vi "configureAcquisition.vi"(6 "imagePaths":path[](array[path]), 7 "saveImages?":bool, 8 "error in (no error)":errorcluster, 9 "number of Images":i32, 10 "CamaraSettings":refnum<class "CamaraSettings.lvclass">, 11 "NetworkWinX32 in":refnum<class "NetworkWinX32.lvclass">) -> (0 "error out":errorcluster, 3 "NetworkWinX32 out":refnum<class "NetworkWinX32.lvclass">)   [LabVIEW 2011, in "Hardware.lvlib" / "HWControllers.lvlib" / "NetworkWinX32.lvclass"]
uses:
  NetworkWinX32.lvclass
  Tools/CameraSettings/CamaraSettings.lvclass
  NetworkWinX32.lvclass/NetworkWinX32.ctl
  Channels/Camera/WinX32_SA/WinX32Camera.lvclass
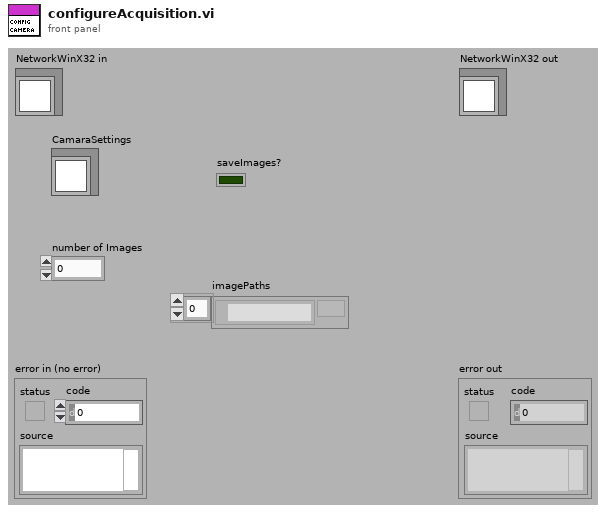
[diagram p1: front panel]
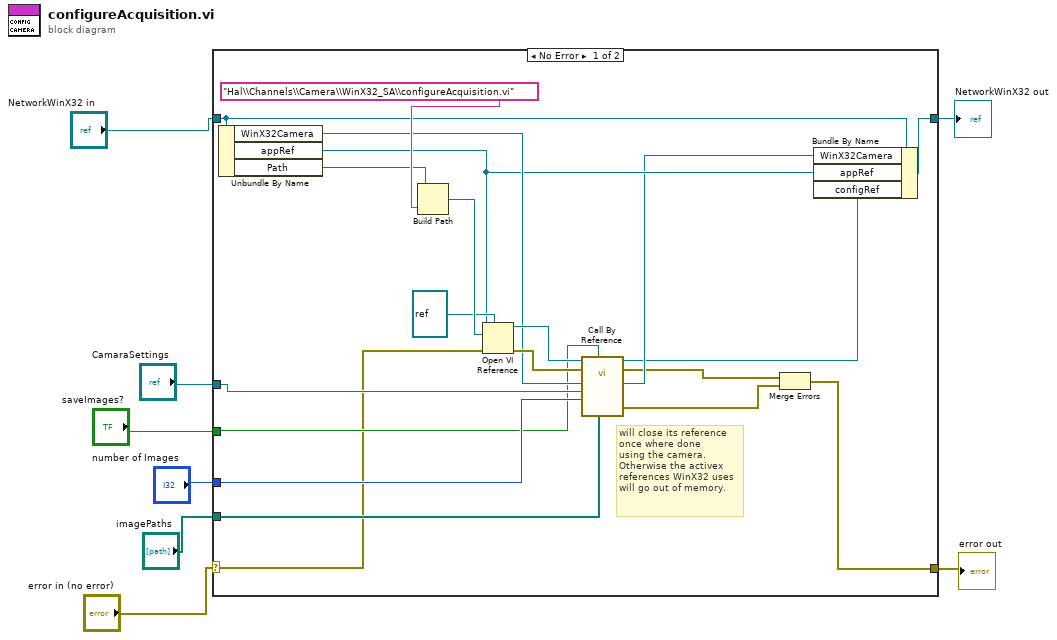
[diagram p0: block diagram]
diagram:
  n1 = case shown="No Error" "error in (no error)" {
    selector: "error in (no error)" -> [w11 w30]
    tunnel: [w12 w30] -> w6
    tunnel: [w13 w29] -> w7
    tunnel: "NetworkWinX32 in" -> [w16 w29]
    tunnel: "CamaraSettings" -> [w22 _]
    tunnel: "saveImages?" -> [w19 _]
    tunnel: "number of Images" -> [w20 _]
    tunnel: "imagePaths" -> [w18 _]
    frame No Error {
      # "will close its reference\nonce where done\nusing the camera.\nOtherwise the activex\nreferences WinX32 uses\nwill go out of memory."
      n2 = Unbundle By Name(w16) -> ("WinX32Camera"=w21:refnum<class "WinX32Camera.lvclass">, "appRef"=w15:refnum<vi>, "Path"=w26:path)
      n3 = Build Path(base path=w26, name or relative path="Hal\\Channels\\Camera\\WinX32_SA\\configureAcquisition.vi" ("viPath")) -> (appended path=w28:path)
      n4 = Open VI Reference(type specifier VI Refnum (for type only)=refnum<vi> refnum, application reference (local)=w15, vi path=w28, error in (no error)=w11) -> (vi reference=w23:refnum<vi>, error out=w24:errorcluster)  [unwired: 2 in]
      n5 = call-by-ref "?"(reference=w23, error in=w24, "imagePaths"=w18, "saveImages?"=w19, "number of Images"=w20, "CameraSettings"=w22, "WinX32Camera in"=w21) -> (reference out=w9:refnum<vi>, error out=w10:errorcluster, 0:"error out"=w17:errorcluster, "WinX32Camera out"=w14:refnum<class "WinX32Camera.lvclass">)  [unwired: 5 in]
      n6 = Merge Errors(w10, w17) -> (w12:errorcluster)
      n7 = Bundle By Name(cluster=w16, "WinX32Camera"=w14, "appRef"=w15, "configRef"=w9) -> (w13:refnum<class "NetworkWinX32.lvclass">)
    }
    frame Error {
    }
  }
  "error out" <- w6
  "NetworkWinX32 out" <- w7
